vi "Write External Launch.vi"(8 "error in (no error)":errorcluster, 10 "External Launch":bool, 11 "NistModuleAdminBase in":refnum<class "ModuleAdminBase.lvclass">) -> (0 "error out":errorcluster, 3 "NistModuleAdminBase out":refnum<class "ModuleAdminBase.lvclass">)   [LabVIEW 2014, in "ModuleAdmin.lvlib" / "ModuleAdminBase.lvclass"]
uses:
  ModuleAdminBase.lvclass
  ModuleAdminBase.lvclass/ModuleAdminBase.ctl
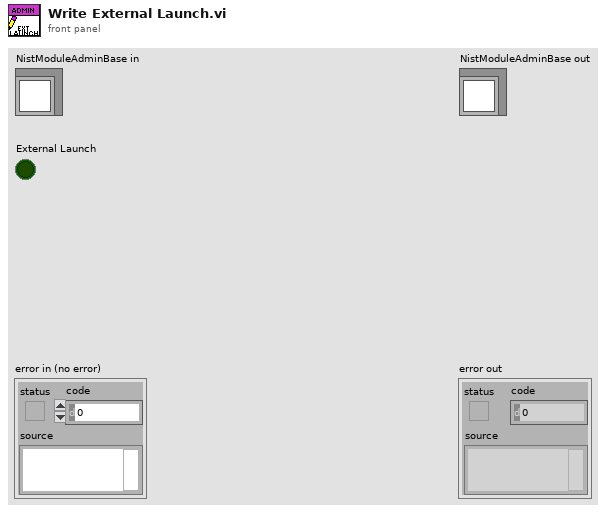
[diagram p1: front panel]
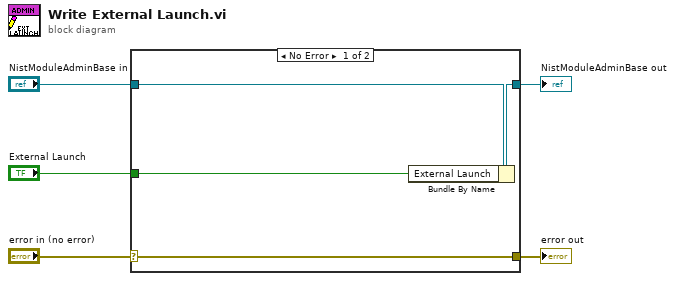
[diagram p0: block diagram]
diagram:
  n1 = case shown="No Error" "error in (no error)" {
    selector: "error in (no error)" -> [w9 w10]
    tunnel: [w9 w10] -> w4
    tunnel: [w7 w11] -> w2
    tunnel: "NistModuleAdminBase in" -> [w8 w11]
    tunnel: "External Launch" -> [w6 _]
    frame No Error {
      n2 = Bundle By Name(cluster=w8, "External Launch"=w6) -> (w7:refnum<class "ModuleAdminBase.lvclass">)
    }
    frame Error {
    }
  }
  "error out" <- w4
  "NistModuleAdminBase out" <- w2
